vi "InitializeGrid.vi"(9 "n vertical":dbl, 10 "n horizontal":dbl, 11 "grid in":T1) -> (2 "grid out":T1)   [LabVIEW 2016]
uses:
  grid.ctl
  elementGrid.ctl
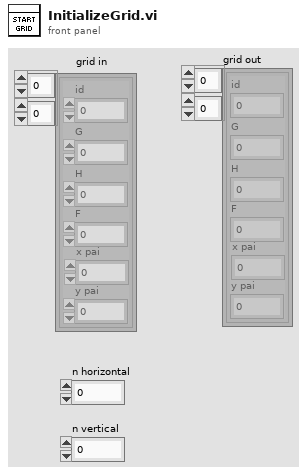
[diagram p1: front panel]
types:
  T1 = typedef "grid.ctl" = T2[][]
  T2 = typedef "elementGrid.ctl" = cluster{"id":dbl, "G":dbl, "H":dbl, "F":dbl, "x pai":dbl, "y pai":dbl}
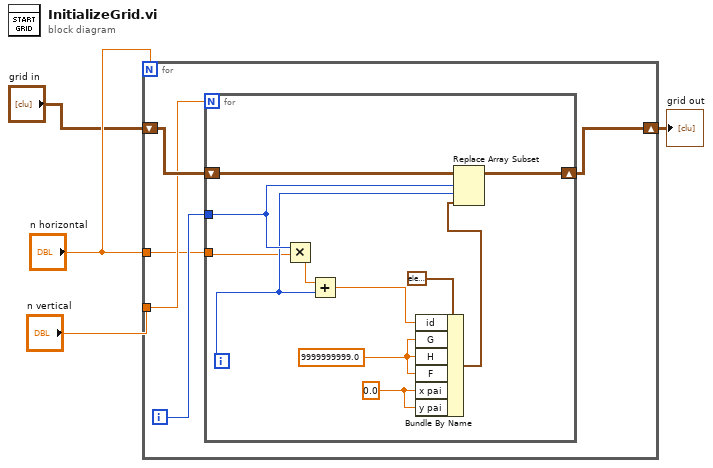
[diagram p0: block diagram]
diagram:
  n1 = for {
    N: "n horizontal" -> [_]
    shift-right: [w7] -> w1
    shift-left: "grid in" -> [w9]
    tunnel: "n vertical" -> [w6]
    tunnel: "n horizontal" -> [w5]
    i -> [w8]
    n2 = for {
      N: w6 -> [_]
      shift-right: [w16] -> w7
      shift-left: w9 -> [w18]
      tunnel: w8 -> [w17]
      tunnel: w5 -> [w13]
      i -> [w15]
      w10 = 0.0 ("x pai")
      w12 = 9999999999.0
      n3 = Multiply(x=w17, y=w13) -> (x*y=w20:dbl)
      n4 = Add(x=w20, y=w15) -> (x+y=w19:dbl)
      n5 = Bundle By Name(cluster=T2 {"id"=0.0, "G"=0.0, "H"=0.0, "F"=0.0, "x pai"=0.0, "y pai"=0.0} ("element"), "id"=w19, "G"=w12, "H"=w12, "F"=w12, "x pai"=w10, "y pai"=w10) -> (w14:T2)
      n6 = Replace Array Subset(array=w18, new element=w14, index (row)=w17, index (col)=w15) -> (w16:T1)
    }
  }
  "grid out" <- w1
